vi "Go Home Position.vi"(8 "error in (no error)":errorcluster, 9 "Rate (Hz)":dbl=1000.0 format="%#_13g", 10 "Velocity factor":dbl=0.5 format="%#_13g", 11 "Grips Robot in":refnum<class "Grips Robot.lvclass">) -> (0 "error out":errorcluster, 1 "Debug":dbl[](array[numeric]), 2 "Joint Positions":dbl[](array[numeric]), 3 "Grips Robot out":refnum<class "Grips Robot.lvclass">)   [LabVIEW 2013, in "Grips Robot.lvclass"]
uses:
  Grips Robot.lvclass
  Grips Robot.lvclass/Grips Robot.ctl
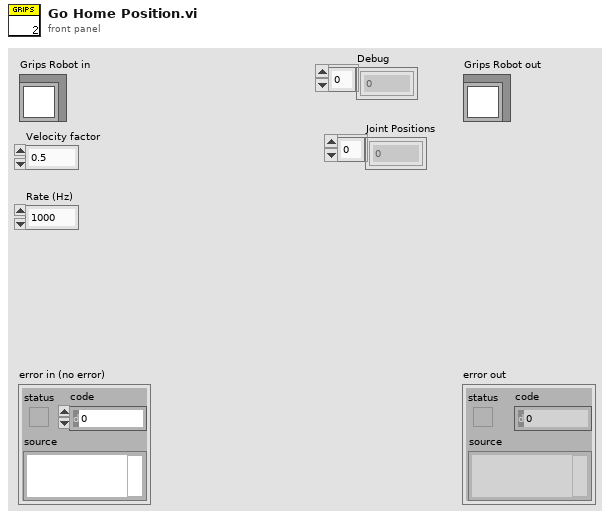
[diagram p1: front panel]
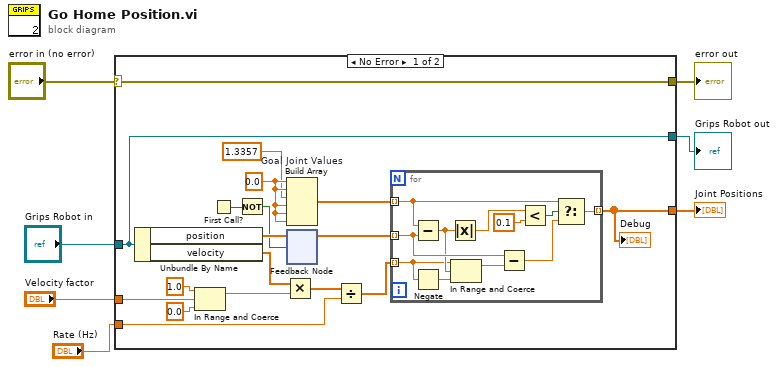
[diagram p0: block diagram]
diagram:
  n1 = case shown="No Error" "error in (no error)" {
    selector: "error in (no error)" -> [w25 w38]
    tunnel: [w25 w38] -> w6
    tunnel: [w24 w37] -> w4
    tunnel: "Grips Robot in" -> [w24 w37]
    tunnel: "Velocity factor" -> [w21 _]
    tunnel: "Rate (Hz)" -> [w15 _]
    tunnel: [w8 _] -> w1
    frame No Error {
      w23 = 0.0 ("element")
      n2 = Unbundle By Name(w24) -> ("position"=w12:dbl[], "velocity"=w18:dbl[])
      n3 = In Range and Coerce(upper limit=1.0, x=w21, lower limit=0.0) -> (coerced(x)=w17:dbl)  [unwired: 1 out]
      n4 = First Call?() -> (First Call?: T/F=w10:bool)
      n5 = Not(x=w10) -> (.not. x?=w9:bool)
      n6 = Multiply(x=w18, y=w17) -> (x*y=w16:dbl[])
      n7 = Build Array "Goal Joint Values"(w23, w23, 1.3357 ("element"), w23, w23, w23) -> (w22:dbl[])
      n8 = feedback-in #1(w12, w9) -> ()
      n9 = feedback #1() -> (w11:dbl[])  [unwired: 1 in]
      n10 = Divide(x=w16, y=w15) -> (x/y=w14:dbl[])
      n11 = for {
        tunnel: w22 -> [w27] mode=indexing
        tunnel: w11 -> [w36] mode=indexing
        tunnel: w14 -> [w29] mode=indexing
        tunnel: [w31] -> w8 mode=indexing
        n12 = Subtract(x=w27, y=w36) -> (x-y=w34:dbl)
        n13 = Negate(x=w29) -> (-x=w35:dbl)
        n14 = Absolute Value(x=w34) -> (abs(x)=w33:dbl)
        n15 = In Range and Coerce(upper limit=w29, x=w34, lower limit=w35) -> (coerced(x)=w30:dbl)  [unwired: 1 out]
        n16 = Subtract(x=w36, y=w30) -> (x-y=w28:dbl)
        n17 = Less?(x=w33, y=0.1) -> (x < y?=w32:bool)
        n18 = Select(t=w27, s=w32, f=w28) -> (s? t:f=w31:dbl)
      }
      "Debug" <- w8
    }
    frame Error {
    }
  }
  "error out" <- w6
  "Grips Robot out" <- w4
  "Joint Positions" <- w1
